vi "ToString.vi"(8 "error in (no error)":errorcluster, 11 "TestSuite In":refnum<class "TestSuite.lvclass">) -> (0 "error out":errorcluster, 2 "String":string, 3 "TestSuite Out":refnum<class "TestSuite.lvclass">)   [LabVIEW 2017, in "TestSuite.lvclass"]
doc: "Returns the string representation for this object."
uses:
  TestSuite.lvclass
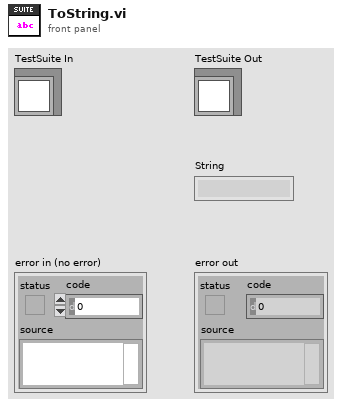
[diagram p1: front panel]
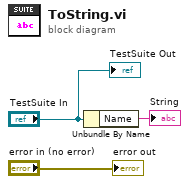
[diagram p0: block diagram]
diagram:
  n1 = Unbundle By Name("TestSuite In") -> ("Name"=→"String":string)
  "error out" <- "error in (no error)"
  "TestSuite Out" <- "TestSuite In"
